vi "WaveFormDecimate_single.vi"(6 "Decimation factor":i32, 7 "Plot interpolation":T1(ring), 8 "error in (no error)":errorcluster, 11 "Waveform in":waveform(dbl)) -> (0 "error out":errorcluster, 3 "Waveform out":waveform(dbl))   [LabVIEW 2015]
uses:
  <vilib>/measure/maresamp.llb/Resample Waveform (single shot).vi
  <vilib>/measure/NI_MAPro.lvlib
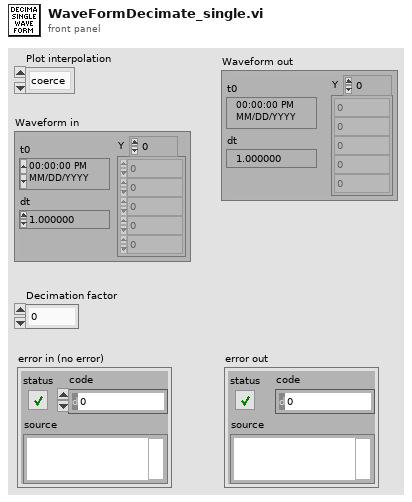
[diagram p1: front panel]
types:
  T1 = enum16{"coerce", "linear", "spline", "Min-Max", "Average"}
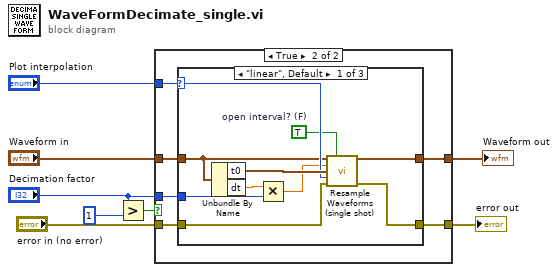
[diagram p0: block diagram]
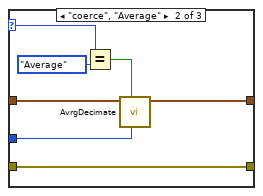
[diagram p3: hidden frame]
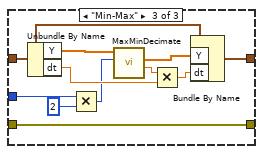
[diagram p4: hidden frame]
diagram:
  n1 = Greater?(x="Decimation factor", y=1) -> (0:w6:bool)
  n2 = case shown="True" w6 {
    tunnel: [w10 w16] -> w1
    tunnel: "Plot interpolation" -> [_ w15]
    tunnel: [w9 w14] -> w3
    tunnel: "error in (no error)" -> [w9 w13]
    tunnel: "Waveform in" -> [w10 w12]
    tunnel: "Decimation factor" -> [_ w11]
    frame False {
    }
    frame True {
      n3 = case shown="\"linear\", Default" w15 {
        selector: w15 -> [w25 w28 _]
        tunnel: w12 -> [w18 w33 w43]
        tunnel: w11 -> [w21 w31 w41]
        tunnel: [w17 w32 w40] -> w16
        tunnel: [w24 w30 w36] -> w14
        tunnel: w13 -> [w23 w30 w36]
        frame "linear", Default {
          w19 = TRUE  # open interval? (F)
          n4 = Unbundle By Name(w18) -> ("t0"=w26:timestamp, "dt"=w22:dbl)
          n5 = Multiply(x=w22, y=w21) -> (x*y=w20:dbl)
          n6 = call-poly <vilib>:"Resample Waveforms (single shot).vi"("waveform in"=w18, "open interval? (F)"=w19, "dt"=w20, "t0"=w26, "interpolation mode"=w25, "error in (no error)"=w23) -> ("resampled waveform out"=w17:waveform(dbl), "error out"=w24:errorcluster)  [unwired: 6 in, 2 out]
        }
        frame "coerce", "Average" {
          n7 = Equal?(x=w28, y=T1."Average" ("Plot interpolation")) -> (x = y?=w27:bool)
          n8 = call "AvrgDecimate.vi"("Decimate by"=w31, "Average?"=w27, "waveform"=w33) -> ("output waveform"=w32:waveform(sgl))  [unwired: 8 out]
        }
        frame "Min-Max" {
          n9 = Unbundle By Name(w43) -> ("Y"=w44:dbl[], "dt"=w37:dbl)
          n10 = Multiply(x=w41, y=2) -> (x*y=w35:i32)
          n11 = call "MaxMinDecimate.vi"("decimation factor"=w35, "Array"=w44) -> ("actual decimation"=w39:sgl, "decimated array"=w42:sgl[])  [unwired: 8 out]
          n12 = Multiply(x=w39, y=w37) -> (x*y=w38:dbl)
          n13 = Bundle By Name(cluster=w43, "Y"=w42, "dt"=w38) -> (w40:waveform(dbl))
        }
      }
    }
  }
  "error out" <- w3
  "Waveform out" <- w1
